vi "terminate.vi"(8 "error in (no error)":errorcluster, 11 "GenericPlugin in":refnum<class "ScanHeadAK130114ResonanceFlexRIO.lvclass">) -> (0 "error out":errorcluster, 3 "GenericPlugin out":refnum<class "ScanHeadAK130114ResonanceFlexRIO.lvclass">)   [LabVIEW 2010, in "ScanHeadAK130114ResonanceFlexRIO.lvclass"]
doc: "The dynamic dispatch version of this VI terminates the plug-in object by releasing all of its resources."
uses:
  ScanHeadAK130114ResonanceFlexRIO.lvclass
  AnalogOut/GenericAnalogOut/GenericAnalogOut/GenericAnalogOut.lvclass
  SignalWriter/GenericSignalWriter/GenericSignalWriter/GenericSignalWriter.lvclass
  GenericScanHead/GenericScanHead/GenericScanHead.lvclass
  common/classes/ErrorController/ErrorController/class_data.vi
  common/classes/ErrorController/ErrorController/ErrorController.lvclass
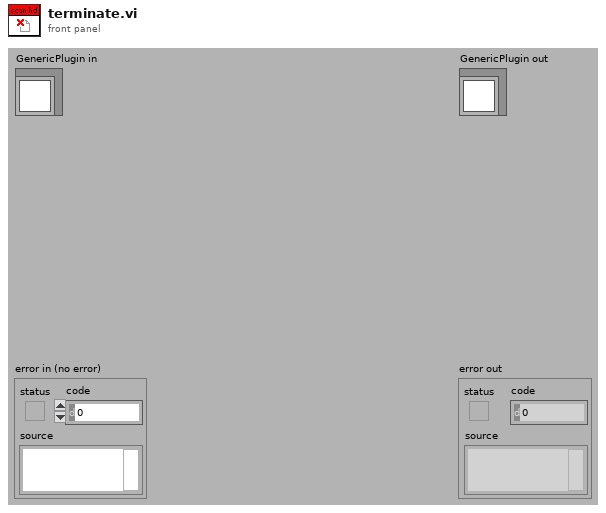
[diagram p1: front panel]
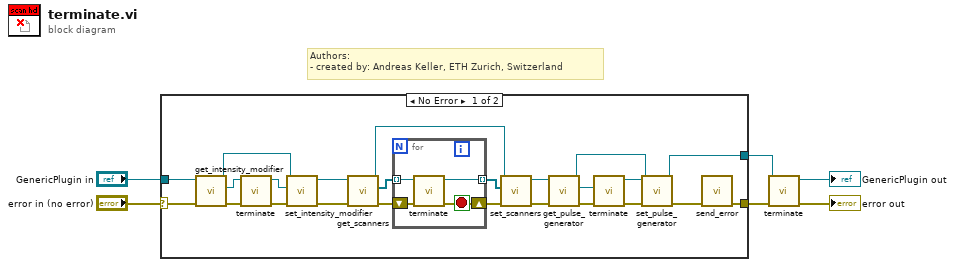
[diagram p0: block diagram]
diagram:
  # "Authors: \n- created by: Andreas Keller, ETH Zurich, Switzerland"
  n1 = case shown="No Error" "error in (no error)" {
    selector: "error in (no error)" -> [w30 w36]
    tunnel: [w7 w35] -> w3
    tunnel: "GenericPlugin in" -> [w25 w35]
    tunnel: [w11 w36] -> w1
    frame No Error {
      n2 = call-dynamic "get_intensity_modifier.vi"("error in (no error)"=w30, "ScanHeadAK130114ResonanceFlexRIO in"=w25) -> ("error out"=w29:errorcluster, "intensity modifier"=w27:refnum<class "GenericAnalogOut.lvclass">, "ScanHeadAK130114ResonanceFlexRIO out"=w24:refnum<class "ScanHeadAK130114ResonanceFlexRIO.lvclass">)  [unwired: 7 in]
      n3 = call-dynamic "terminate.vi"("error in (no error)"=w29, "GenericPlugin in"=w27) -> ("error out"=w28:errorcluster, "GenericPlugin out"=w26:refnum<class "GenericAnalogOut.lvclass">)  [unwired: 8 in]
      n4 = call-dynamic "set_intensity_modifier.vi"("error in (no error)"=w28, "intensity modifier"=w26, "ScanHeadAK130114ResonanceFlexRIO in"=w24) -> ("error out"=w23:errorcluster, "ScanHeadAK130114ResonanceFlexRIO out"=w22:refnum<class "ScanHeadAK130114ResonanceFlexRIO.lvclass">)  [unwired: 7 in]
      n5 = call-dynamic "get_scanners.vi"("error in (no error)"=w23, "ScanHeadAK130114ResonanceFlexRIO in"=w22) -> ("error out"=w20:errorcluster, "scanners"=w19:refnum<class "GenericSignalWriter.lvclass">[], "ScanHeadAK130114ResonanceFlexRIO out"=w21:refnum<class "ScanHeadAK130114ResonanceFlexRIO.lvclass">)  [unwired: 7 in]
      n6 = for {
        shift-right: [w31] -> w17
        shift-left: w20 -> [w32]
        tunnel: w19 -> [w34] mode=indexing
        tunnel: [w33] -> w18 mode=indexing
        stop <- w31 stop-if-true
        n7 = call-dynamic "terminate.vi"("error in (no error)"=w32, "GenericPlugin in"=w34) -> ("error out"=w31:errorcluster, "GenericPlugin out"=w33:refnum<class "GenericSignalWriter.lvclass">)  [unwired: 8 in]
      }
      n8 = call-dynamic "set_scanners.vi"("error in (no error)"=w17, "scanners"=w18, "ScanHeadAK130114ResonanceFlexRIO in"=w21) -> ("error out"=w16:errorcluster, "ScanHeadAK130114ResonanceFlexRIO out"=w15:refnum<class "ScanHeadAK130114ResonanceFlexRIO.lvclass">)  [unwired: 7 in]
      n9 = call-dynamic "get_pulse_generator.vi"("error in (no error)"=w16, "ScanHeadAK130114ResonanceFlexRIO in"=w15) -> ("error out"=w14:errorcluster, "pulse generator"=w10:refnum<class "GenericSignalWriter.lvclass">, "ScanHeadAK130114ResonanceFlexRIO out"=w8:refnum<class "ScanHeadAK130114ResonanceFlexRIO.lvclass">)  [unwired: 7 in]
      n10 = call-dynamic "terminate.vi"("error in (no error)"=w14, "GenericPlugin in"=w10) -> ("error out"=w13:errorcluster, "GenericPlugin out"=w9:refnum<class "GenericSignalWriter.lvclass">)  [unwired: 8 in]
      n11 = call-dynamic "set_pulse_generator.vi"("error in (no error)"=w13, "pulse generator"=w9, "ScanHeadAK130114ResonanceFlexRIO in"=w8) -> ("error out"=w12:errorcluster, "ScanHeadAK130114ResonanceFlexRIO out"=w7:refnum<class "ScanHeadAK130114ResonanceFlexRIO.lvclass">)  [unwired: 7 in]
      n12 = call "send_error.vi"("error in (no error)"=w12) -> ("error out"=w11:errorcluster)  [unwired: 10 in]
    }
    frame Error {
    }
  }
  n13 = call-parent "terminate.vi"("error in (no error)"=w1, "GenericPlugin in"=w3) -> ("error out"=→"error out":errorcluster, "GenericPlugin out"=→"GenericPlugin out":refnum<class "ScanHeadAK130114ResonanceFlexRIO.lvclass">)  [unwired: 8 in]
